vi "Shutdown Daemon.vi"(8 "error in (no error)":errorcluster, 11 "TCP slave in":refnum<class "TCP Slave.lvclass">) -> (0 "error out":errorcluster)   [LabVIEW 2015, in "SubVIs.lvlib" / "TCP Slave.lvclass"]
doc: "Sends a notification to the daemon and connection handlers, commanding them to quit."
uses:
  <vilib>/Modbus/subvis/Protocol/TCP/TCP Slave/TCP Slave.lvclass
  <vilib>/Modbus/subvis/Protocol/TCP/TCP Slave/TCP Slave.lvclass/TCP Slave.ctl
  <vilib>/Modbus/subvis/Protocol/Interfaces/Network Slave/Network Slave.lvclass
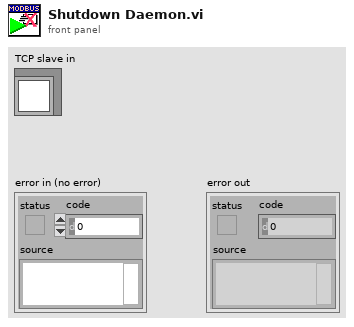
[diagram p1: front panel]
types:
  T1 = typedef "SubVIs.lvlib/TCP Slave.lvclass/Connection Counter.ctl" = cluster{"Currently Connected":u32, "Connection Records":refnum<data-value>[]}
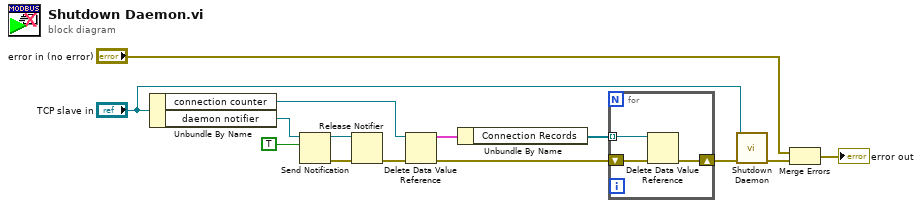
[diagram p0: block diagram]
diagram:
  n1 = Unbundle By Name("TCP slave in") -> ("connection counter"=w8:refnum<data-value>, "daemon notifier"=w11:refnum<notifier>)
  n2 = Send Notification(notification=TRUE, notifier=w11) -> (notifier out=w13:refnum<notifier>, error out=w12:errorcluster)  [unwired: 1 in]
  n3 = Release Notifier(notifier=w13, error in (no error)=w12) -> (error out=w9:errorcluster)  [unwired: 1 in, 2 out]
  n4 = Delete Data Value Reference(data value reference=w8, error in=w9) -> (data value=w5:T1, error out=w7:errorcluster)
  n5 = Unbundle By Name(w5) -> ("Connection Records"=w4:refnum<data-value>[])
  n6 = for {
    shift-right: [w15] -> w6
    shift-left: w7 -> [w16]
    tunnel: w4 -> [w17] mode=indexing
    n7 = Delete Data Value Reference(data value reference=w17, error in=w16) -> (error out=w15:errorcluster)  [unwired: 1 out]
  }
  n8 = call-parent "Shutdown Daemon.vi"("error in (no error)"=w6, "network slave in"="TCP slave in") -> ("error out"=w2:errorcluster)  [unwired: 9 in]
  n9 = Merge Errors("error in (no error)", w2) -> (→"error out":errorcluster)
